vi "test_libssh2_channel_forward_accept.vi"() -> ()   [LabVIEW 2017, in "integration_tests.lvlib"]
uses:
  integration_tests.lvlib
  libssh2/libssh2_channel_forward_listen_ex.vi
  support/support.lvlib
  libssh2/libssh2.lvlib
  <vilib>/PNR/Transparent Assertions/Transparent Assertions/Transparent Assertions.lvlib
panel:
  out "error out":errorcluster
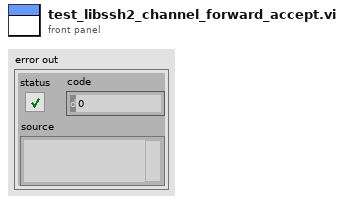
[diagram p1: front panel]
types:
  T1 = typedef "libssh2.lvlib/Session Refnum.ctl" = refnum<k1>
  T2 = typedef "libssh2.lvlib/Listener Refnum.ctl" = refnum<k1>
  T3 = typedef "libssh2.lvlib/Channel Refnum.ctl" = refnum<k1>
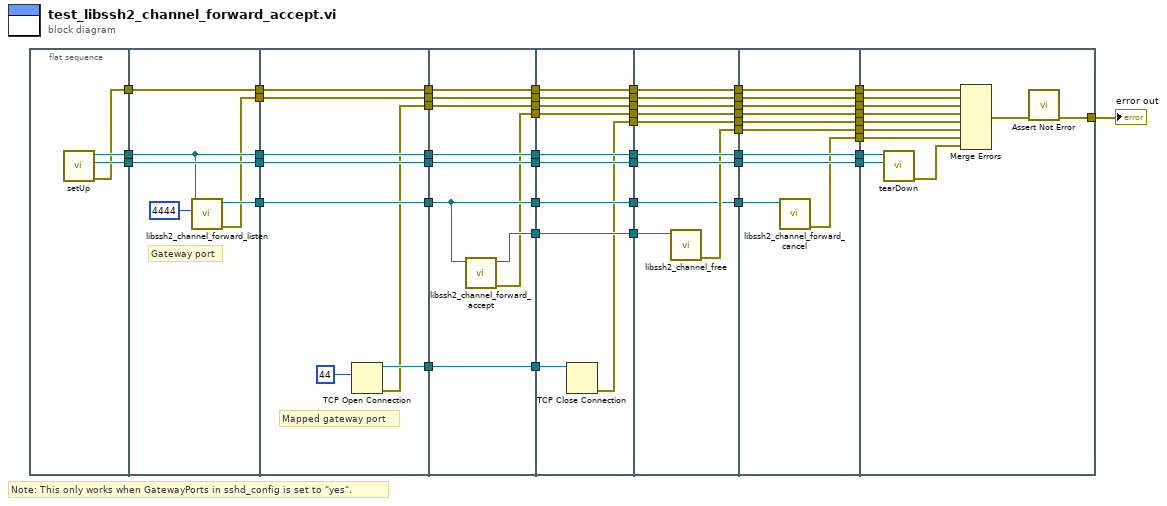
[diagram p0: block diagram]
diagram:
  # "Note: This only works when GatewayPorts in sshd_config is set to \"yes\"."
  n1 = flat-sequence {
    tunnel: [w55] -> w52
    tunnel: [w54] -> w51
    tunnel: [w53] -> w50
    tunnel: w52 -> [w59]
    tunnel: w51 -> [w61]
    tunnel: [w59] -> w35
    tunnel: [w61] -> w33
    tunnel: w50 -> [w60]
    tunnel: [w60] -> w31
    tunnel: [w57] -> w29
    tunnel: [w58] -> w27
    tunnel: w35 -> [w65]
    tunnel: [w65] -> w34
    tunnel: w33 -> [w69]
    tunnel: [w69] -> w32
    tunnel: w31 -> [w68]
    tunnel: [w68] -> w30
    tunnel: w29 -> [w67]
    tunnel: [w67] -> w28
    tunnel: w27 -> [w66]
    tunnel: [w66] -> w26
    tunnel: [w63] -> w25
    tunnel: [w62] -> w24
    tunnel: w34 -> [w78]
    tunnel: [w78] -> w43
    tunnel: w32 -> [w77]
    tunnel: [w77] -> w42
    tunnel: w30 -> [w76]
    tunnel: [w76] -> w41
    tunnel: w28 -> [w75]
    tunnel: [w75] -> w40
    tunnel: w26 -> [w74]
    tunnel: [w74] -> w39
    tunnel: [w73] -> w38
    tunnel: [w72] -> w37
    tunnel: w25 -> [w72]
    tunnel: w24 -> [w71]
    tunnel: [w71] -> w23
    tunnel: [w70] -> w4
    tunnel: w43 -> [w88]
    tunnel: w42 -> [w87]
    tunnel: [w88] -> w49
    tunnel: [w87] -> w48
    tunnel: [w84] -> w47
    tunnel: w41 -> [w86]
    tunnel: [w86] -> w46
    tunnel: w40 -> [w85]
    tunnel: [w85] -> w45
    tunnel: w39 -> [w82]
    tunnel: w38 -> [w84]
    tunnel: w37 -> [w83]
    tunnel: [w82] -> w36
    tunnel: w23 -> [w81]
    tunnel: [w81] -> w22
    tunnel: [w80] -> w21
    tunnel: w4 -> [w79]
    tunnel: [w79] -> w3
    tunnel: w49 -> [w98]
    tunnel: w48 -> [w97]
    tunnel: w47 -> [w96]
    tunnel: [w98] -> w20
    tunnel: [w97] -> w18
    tunnel: [w95] -> w16
    tunnel: w46 -> [w94]
    tunnel: [w94] -> w14
    tunnel: w45 -> [w93]
    tunnel: [w93] -> w12
    tunnel: [w92] -> w10
    tunnel: w36 -> [w92]
    tunnel: w22 -> [w91]
    tunnel: [w91] -> w9
    tunnel: w21 -> [w90]
    tunnel: [w90] -> w7
    tunnel: w3 -> [w89]
    tunnel: [w89] -> w2
    tunnel: w20 -> [w108]
    tunnel: [w108] -> w19
    tunnel: w18 -> [w107]
    tunnel: [w107] -> w17
    tunnel: w16 -> [w106]
    tunnel: [w106] -> w15
    tunnel: w14 -> [w105]
    tunnel: [w105] -> w13
    tunnel: w12 -> [w104]
    tunnel: [w104] -> w11
    tunnel: w10 -> [w101]
    tunnel: w9 -> [w103]
    tunnel: [w103] -> w8
    tunnel: w7 -> [w102]
    tunnel: [w102] -> w6
    tunnel: [w100] -> w5
    tunnel: w2 -> [w99]
    tunnel: [w99] -> w1
    tunnel: w19 -> [w120]
    tunnel: w17 -> [w119]
    tunnel: [w118] -> w44
    tunnel: w15 -> [w116]
    tunnel: w13 -> [w115]
    tunnel: w11 -> [w113]
    tunnel: w8 -> [w112]
    tunnel: w6 -> [w111]
    tunnel: w5 -> [w110]
    tunnel: w1 -> [w109]
    frame #0 {
      n2 = call "setUp.vi"() -> ("error out"=w53:errorcluster, "connection ID"=w54:refnum<k5>, "session"=w55:T1)  [unwired: 9 in]
    }
    frame #1 {
      # "Gateway port"
      n3 = call "libssh2_channel_forward_listen.vi"("port in"=4444, "session"=w59) -> ("error out"=w57:errorcluster, "listener"=w58:T2)  [unwired: 7 in, 1 out]
    }
    frame #2 {
      # "Mapped gateway port"
      n4 = TCP Open Connection(remote port or service name=u16 44) -> (connection ID=w63:refnum<k5>, error out=w62:errorcluster)  [unwired: 4 in]
    }
    frame #3 {
      n5 = call "libssh2_channel_forward_accept.vi"("listener"=w74) -> ("error out"=w70:errorcluster, "channel"=w73:T3)  [unwired: 9 in]
    }
    frame #4 {
      n6 = TCP Close Connection(connection ID=w83) -> (error out=w80:errorcluster)  [unwired: 2 in, 1 out]
    }
    frame #5 {
      n7 = call "libssh2_channel_free.vi"("channel"=w96) -> ("error out"=w95:errorcluster)  [unwired: 10 in]
    }
    frame #6 {
      n8 = call "libssh2_channel_forward_cancel.vi"("listener"=w101) -> ("error out"=w100:errorcluster)  [unwired: 10 in]
    }
    frame #7 {
      n9 = call "tearDown.vi"("connection ID"=w119, "session"=w120) -> ("error out"=w117:errorcluster)  [unwired: 9 in]
      n10 = Merge Errors(w115, w113, w112, w109, w111, w116, w110, w117) -> (w114:errorcluster)
      n11 = call <vilib>:"Assert Not Error.vi"("error in (no error)"=w114) -> ("error out"=w118:errorcluster)  [unwired: 10 in]
    }
  }
  "error out" <- w44
